vi "Stop.vi"   [LabVIEW 2014]
uses:
  Application/SmartPalette/Palette.vi
  Application/SmartPalette/SmartPalette.lvlib
types:
  T1 = enum32{"Invalid", "Standard", "Closed", "Hidden", "Minimized", "Maximized"}
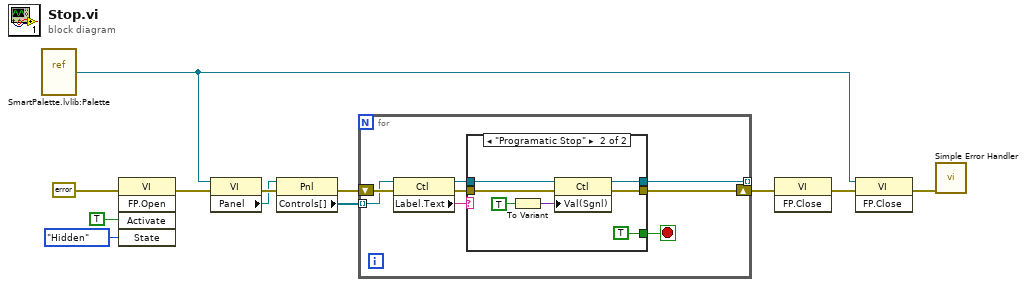
[diagram p0: block diagram]
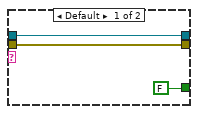
[diagram p2: hidden frame]
diagram:
  n1 = vi-ref "SmartPalette.lvlib:Palette.vi"() -> (w5:refnum<vi>)
  n2 = invoke class="VI" method="FP.Open"(error in=errorcluster {"status"=FALSE, "code"=0, "source"=""} ("error constant"), "Activate"=TRUE, "State"=T1."Hidden") -> (error out=w3:errorcluster)  [unwired: 2 in, 4 out]
  n3 = property class="VI"(reference=w5, error in=w3) -> (error out=w12:errorcluster, "Panel"=w11:refnum<vi>)  [unwired: 1 out]
  n4 = property class="Pnl"(reference=w11, error in=w12) -> (error out=w9:errorcluster, "Controls[]"=w10:refnum<vi>[])  [unwired: 1 out]
  n5 = for {
    tunnel: w10 -> [w19] mode=indexing
    shift-right: [w13] -> w8
    shift-left: w9 -> [w20]
    tunnel: [w15] -> _ mode=indexing
    stop <- w17 stop-if-true
    n6 = property class="Ctl"(reference=w19, error in=w20) -> (reference out=w16:refnum<vi>, error out=w14:errorcluster, "Label.Text"=w18:string)
    n7 = case shown="\"Programatic Stop\"" w18 {
      tunnel: [FALSE TRUE] -> w17
      tunnel: w16 -> [w23 w29]
      tunnel: [w23 w27] -> w15
      tunnel: w14 -> [w22 w28]
      tunnel: [w22 w26] -> w13
      frame Default {
      }
      frame "Programatic Stop" {
        n8 = To Variant(anything=TRUE) -> (Variant=w25:variant)
        n9 = property class="Ctl"(reference=w29, error in=w28, "Val(Sgnl)"=w25) -> (reference out=w27:refnum<vi>, error out=w26:errorcluster)
      }
    }
  }
  n10 = invoke class="VI" method="FP.Close"(error in=w8) -> (error out=w7:errorcluster)  [unwired: 2 in, 2 out]
  n11 = invoke class="VI" method="FP.Close"(reference=w5, error in=w7) -> (error out=w6:errorcluster)  [unwired: 1 in, 2 out]
  n12 = call <vilib>:"Simple Error Handler.vi"("error in (no error)"=w6) -> ()  [unwired: 4 in, 5 out]
